vi "Instrument Sequence Data.vi"() -> (0 "Instrument Sequence Data":T1)   [LabVIEW 2014]
uses:
  Instrument Sequence Data.ctl
  Instrument Sequence Config.ctl
  Instrument Sequence Refnums.ctl
  Action.ctl
  Instrument List.ctl
  Plot Data/Electrical Data Plot Refnums.ctl
panel:
  # "LICENSED MATERIALS – PROPERTY OF IBM\nCopyright IBM Corp. 2016,\nALL RIGHTS RESERVED"
  # "LICENSED MATERIALS – PROPERTY OF IBM\nCopyright IBM Corp. 2016, 2016\nALL RIGHTS RESERVED"
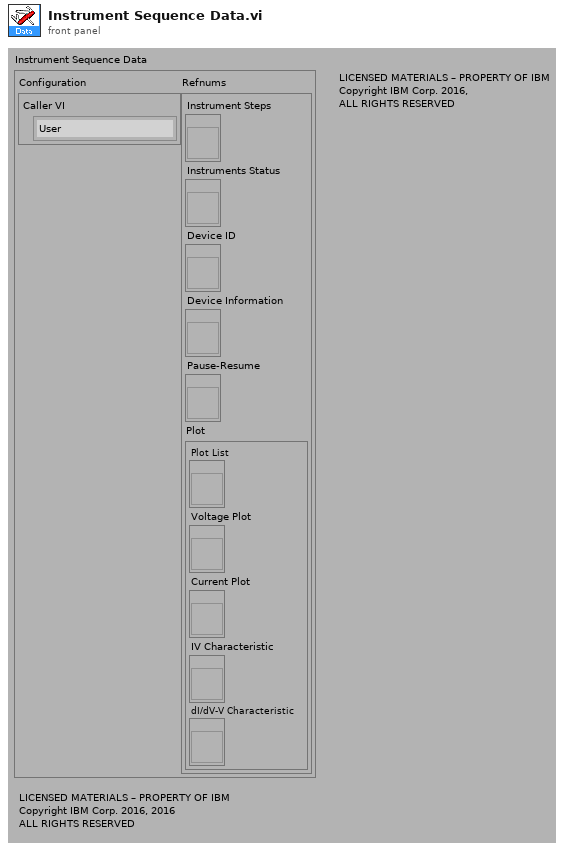
[diagram p1: front panel]
types:
  T1 = typedef "Instrument Sequence Data.ctl" = cluster{"Configuration":T2, "Refnums":T3}
  T2 = typedef "Instrument Sequence Config.ctl" = cluster{"Caller VI":enum16{"User", "Stress Measurement VI"}}
  T3 = typedef "Instrument Sequence Refnums.ctl" = cluster{"Instrument Steps":refnum<vi>, "Instruments Status":refnum<vi>, "Device ID":refnum<vi>, "Device Information":refnum<vi>, "Pause-Resume":refnum<vi>, "Plot":T4}
  T4 = typedef "Electrical Data Plot Refnums.ctl" = cluster{"Plot List":refnum<vi>, "Voltage Plot":refnum<vi>, "Current Plot":refnum<vi>, "IV Characteristic":refnum<vi>, "dI/dV-V Characteristic":refnum<vi>}
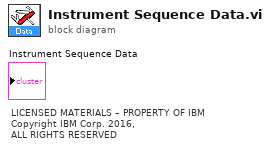
[diagram p0: block diagram]
diagram:
  # "LICENSED MATERIALS – PROPERTY OF IBM\nCopyright IBM Corp. 2016,\nALL RIGHTS RESERVED"
